vi "Read IndexInList.vi"(8 "error in (no error)":errorcluster, 11 "TestMeasureStep in":refnum<class "TestMeasureStep.lvclass">) -> (0 "error out":errorcluster, 2 "IndexInList":u32, 3 "TestMeasureStep out":refnum<class "TestMeasureStep.lvclass">)   [LabVIEW 2017, in "TestMeasureStep.lvclass"]
uses:
  TestMeasureStep.lvclass
  TestMeasureStep.lvclass/TestMeasureStep.ctl
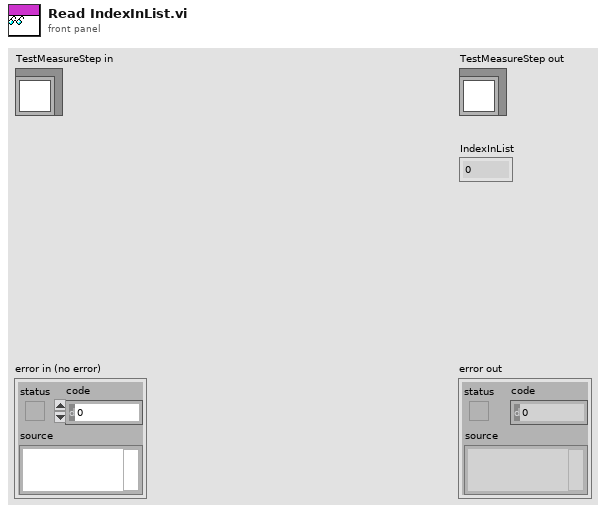
[diagram p1: front panel]
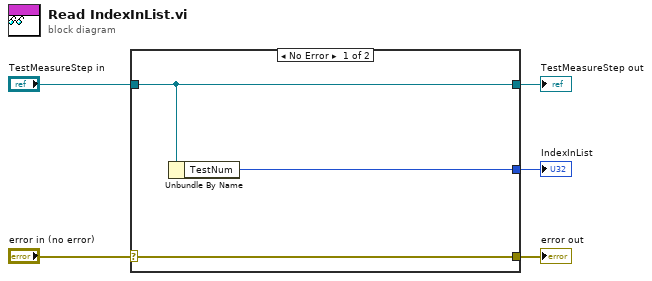
[diagram p0: block diagram]
diagram:
  n1 = case shown="No Error" "error in (no error)" {
    selector: "error in (no error)" -> [w8 w9]
    tunnel: [w8 w9] -> w4
    tunnel: [w7 w10] -> w2
    tunnel: "TestMeasureStep in" -> [w7 w10]
    tunnel: [w6 _] -> w1
    frame No Error {
      n2 = Unbundle By Name(w7) -> ("TestNum"=w6:u32)
    }
    frame Error {
    }
  }
  "error out" <- w4
  "TestMeasureStep out" <- w2
  "IndexInList" <- w1
